vi "WebView2 Init.vi"(8 "error in (no error)":errorcluster, 10 "WebView2 Control":refnum<class "WebView2 Control.lvclass">, 11 "WebView2 Event Filter Interface in":refnum<class "WebView2 Event Filter Interface.lvclass">) -> (0 "error out":errorcluster, 3 "WebView2 Event Filter Interface out":refnum<class "WebView2 Event Filter Interface.lvclass">)   [LabVIEW 2025, in "WebView2.lvlib" / "WebView2 Event Filter Interface.lvclass"]
uses:
  WebView2 Event Filter Interface.lvclass
  WebView2 Control Object/WebView2 Control.lvclass
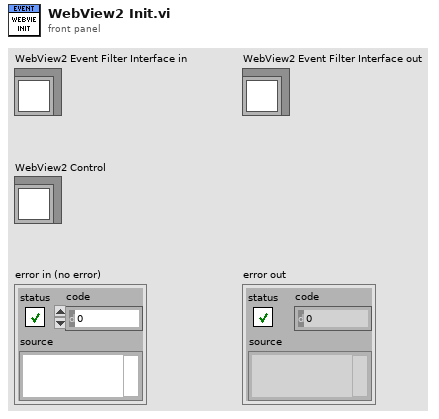
[diagram p1: front panel]
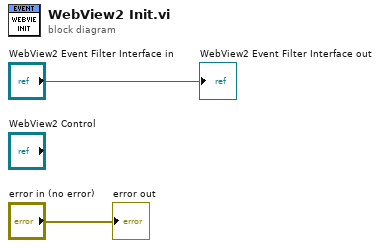
[diagram p0: block diagram]
diagram:
  "error out" <- "error in (no error)"
  "WebView2 Event Filter Interface out" <- "WebView2 Event Filter Interface in"
